vi "Autonomous Independent.vi"() -> ()   [LabVIEW 2016]
doc: "This VI is called when autonomous begins, and will automatically be terminated when autonomous ends. You can carry out timed or sensor driven robot movement independently without needing to return to the caller."
uses:
  2_8_17/Auto_Action.ctl
  <vilib>/Rock Robotics/Network Tables/NT Read Number.vi
  2_11_17/Systems/Global 1.vi
panel:
  out "Auto Mode":dbl=7.0
  in  "Auton_Modes":T2(array[cluster])=[{"Actions"=[{"Effort"=0.55, "Duration"=3.5, "Action"=enum."Nothing", "Encoder"=0.0, "Condition"=FALSE}, {"Effort"=0.0, "Duration"=0.0, "Action"=enum."Nothing", "Encoder"=0.0, "Condition"=FALSE}]}, {"Actions"=[{"Effort"=0.0, "Duration"=0.1, "Action"=enum."Gear1", "Encoder"=6.462, "Condition"=FALSE}, {"Effort"=0.0, "Duration"=0.1, "Action"=enum."Nothing", "Encoder"=0.0, "Condition"=FALSE}, {"Effort"=0.25, "Duration"=1.0, "Action"=enum."Nothing", "Encoder"=38.0, "Condition"=FALSE}, {"Effort"=0.0, "Duration"=0.1, "Action"=enum."Nothing", "Encoder"=0.0, "Condition"=FALSE}, {"Effort"=0.25, "Duration"=0.0, "Action"=enum."Nothing", "Encoder"=57.0, "Condition"=FALSE}, {"Effort"=-0.25, "Duration"=0.0, "Action"=enum."Nothing", "Encoder"=0.0, "Condition"=FALSE}, {"Effort"=1.0, "Duration"=0.0, "Action"=enum."Nothing", "Encoder"=0.0, "Condition"=FALSE}, {"Effort"=0.25, "Duration"=0.0, "Action"=enum."Nothing", "Encoder"=0.0, "Condition"=FALSE}]}, {"Actions"=[{"Effort"=0.0, "Duration"=0.1, "Action"=enum."Drive Encoder Reset", "Encoder"=0.0, "Condition"=FALSE}, {"Effort"=0.0, "Duration"=1.0, "Action"=enum."Gyro Reset", "Encoder"=0.0, "Condition"=FALSE}, {"Effort"=0.3, "Duration"=2.0, "Action"=enum."Drive", "Encoder"=88.0, "Condition"=TRUE}, {"Effort"=1.0, "Duration"=1.0, "Action"=enum."Gear0", "Encoder"=0.0, "Condition"=FALSE}, {"Effort"=1.0, "Duration"=1.0, "Action"=enum."Gear0", "Encoder"=0.0, "Condition"=FALSE}, {"Effort"=1.0, "Duration"=0.5, "Action"=enum."Nothing", "Encoder"=0.0, "Condition"=FALSE}, {"Effort"=0.0, "Duration"=0.0, "Action"=enum."Drive Encoder Reset", "Encoder"=0.0, "Condition"=FALSE}, {"Effort"=0.3, "Duration"=0.5, "Action"=enum."Nothing", "Encoder"=24.0, "Condition"=TRUE}, {"Effort"=0.0, "Duration"=0.0, "Action"=enum."Nothing", "Encoder"=0.0, "Condition"=FALSE}, {"Effort"=-0.2, "Duration"=0.75, "Action"=enum."Drive", "Encoder"=24.0, "Condition"=FALSE}, {"Effort"=0.0, "Duration"=0.0, "Action"=enum."Drive Encoder Reset", "Encoder"=0.0, "Condition"=FALSE}, {"Effort"=-0.25, "Duration"=0.0, "Action"=enum."Nothing", "Encoder"=12.0, "Condition"=FALSE}]}, {"Actions"=[{"Effort"=0.0, "Duration"=0.1, "Action"=enum."Drive Encoder Reset", "Encoder"=6.462, "Condition"=FALSE}, {"Effort"=0.0, "Duration"=0.1, "Action"=enum."Gyro Reset", "Encoder"=0.0, "Condition"=FALSE}, {"Effort"=-0.25, "Duration"=1.0, "Action"=enum."Drive", "Encoder"=6.462, "Condition"=FALSE}, {"Effort"=0.0, "Duration"=0.1, "Action"=enum."Gyro Reset", "Encoder"=0.0, "Condition"=FALSE}, {"Effort"=-0.25, "Duration"=0.0, "Action"=enum."Turn", "Encoder"=57.0, "Condition"=FALSE}, {"Effort"=-0.25, "Duration"=0.0, "Action"=enum."Drive", "Encoder"=7.5, "Condition"=FALSE}, {"Effort"=-1.0, "Duration"=0.0, "Action"=enum."Gear0", "Encoder"=0.0, "Condition"=FALSE}, {"Effort"=0.25, "Duration"=0.0, "Action"=enum."Drive", "Encoder"=3.0, "Condition"=FALSE}]}, {"Actions"=[{"Effort"=0.0, "Duration"=0.1, "Action"=enum."Drive Encoder Reset", "Encoder"=6.462, "Condition"=FALSE}, {"Effort"=0.0, "Duration"=0.1, "Action"=enum."Gyro Reset", "Encoder"=0.0, "Condition"=FALSE}, {"Effort"=-0.25, "Duration"=1.0, "Action"=enum."Drive", "Encoder"=6.462, "Condition"=FALSE}, {"Effort"=0.0, "Duration"=0.1, "Action"=enum."Gyro Reset", "Encoder"=0.0, "Condition"=FALSE}, {"Effort"=-0.25, "Duration"=0.0, "Action"=enum."Turn", "Encoder"=57.0, "Condition"=FALSE}, {"Effort"=-0.25, "Duration"=0.0, "Action"=enum."Drive", "Encoder"=7.5, "Condition"=FALSE}, {"Effort"=-1.0, "Duration"=0.0, "Action"=enum."Gear0", "Encoder"=0.0, "Condition"=FALSE}, {"Effort"=0.25, "Duration"=0.0, "Action"=enum."Drive", "Encoder"=3.0, "Condition"=FALSE}]}, {"Actions"=[{"Effort"=0.0, "Duration"=0.1, "Action"=enum."Drive Encoder Reset", "Encoder"=0.0, "Condition"=FALSE}, {"Effort"=0.0, "Duration"=0.1, "Action"=enum."Gyro Reset", "Encoder"=0.0, "Condition"=FALSE}, {"Effort"=0.25, "Duration"=1.0, "Action"=enum."Drive", "Encoder"=6.462, "Condition"=FALSE}, {"Effort"=1.0, "Duration"=0.1, "Action"=enum."Gyro Reset", "Encoder"=0.0, "Condition"=FALSE}, {"Effort"=0.25, "Duration"=0.0, "Action"=enum."Turn", "Encoder"=57.0, "Condition"=FALSE}, {"Effort"=0.25, "Duration"=0.0, "Action"=enum."Drive", "Encoder"=7.5, "Condition"=FALSE}, {"Effort"=1.0, "Duration"=0.0, "Action"=enum."Gear0", "Encoder"=0.0, "Condition"=FALSE}, {"Effort"=-0.25, "Duration"=0.0, "Action"=enum."Drive", "Encoder"=3.0, "Condition"=FALSE}]}, {"Actions"=[{"Effort"=0.0, "Duration"=0.1, "Action"=enum."Drive Encoder Reset", "Encoder"=0.0, "Condition"=FALSE}, {"Effort"=0.0, "Duration"=0.1, "Action"=enum."Gyro Reset", "Encoder"=0.0, "Condition"=FALSE}, {"Effort"=0.25, "Duration"=5.0, "Action"=enum."Drive", "Encoder"=60000.0, "Condition"=TRUE}, {"Effort"=0.75, "Duration"=1.0, "Action"=enum."Nothing", "Encoder"=0.0, "Condition"=FALSE}, {"Effort"=0.0, "Duration"=1.0, "Action"=enum."Nothing", "Encoder"=0.0, "Condition"=FALSE}, {"Effort"=0.0, "Duration"=0.0, "Action"=enum."Nothing", "Encoder"=0.0, "Condition"=FALSE}]}, {"Actions"=[{"Effort"=0.0, "Duration"=0.5, "Action"=enum."Drive Encoder Reset", "Encoder"=0.0, "Condition"=FALSE}, {"Effort"=0.55, "Duration"=4.25, "Action"=enum."Gyro Reset", "Encoder"=0.0, "Condition"=FALSE}, {"Effort"=0.3, "Duration"=0.0, "Action"=enum."Drive", "Encoder"=60.0, "Condition"=FALSE}, {"Effort"=0.25, "Duration"=1.5, "Action"=enum."Turn", "Encoder"=0.0, "Condition"=FALSE}, {"Effort"=0.25, "Duration"=2.0, "Action"=enum."Vision Correction", "Encoder"=76.6, "Condition"=FALSE}, {"Effort"=0.3, "Duration"=0.5, "Action"=enum."Drive", "Encoder"=0.0, "Condition"=TRUE}]}, {"Actions"=[{"Effort"=0.0, "Duration"=0.0, "Action"=enum."Nothing", "Encoder"=0.0, "Condition"=FALSE}]}]
  # "Nothing"
  # "Boiler Right Right side gear"
  # "Middle Gear"
  # "Boiler Right Left Side Gear"
  # "Boiler Left RightSide Gear"
  # "Boiler Left Left Side Gear"
  # "Drive"
  # "Vision Correction"
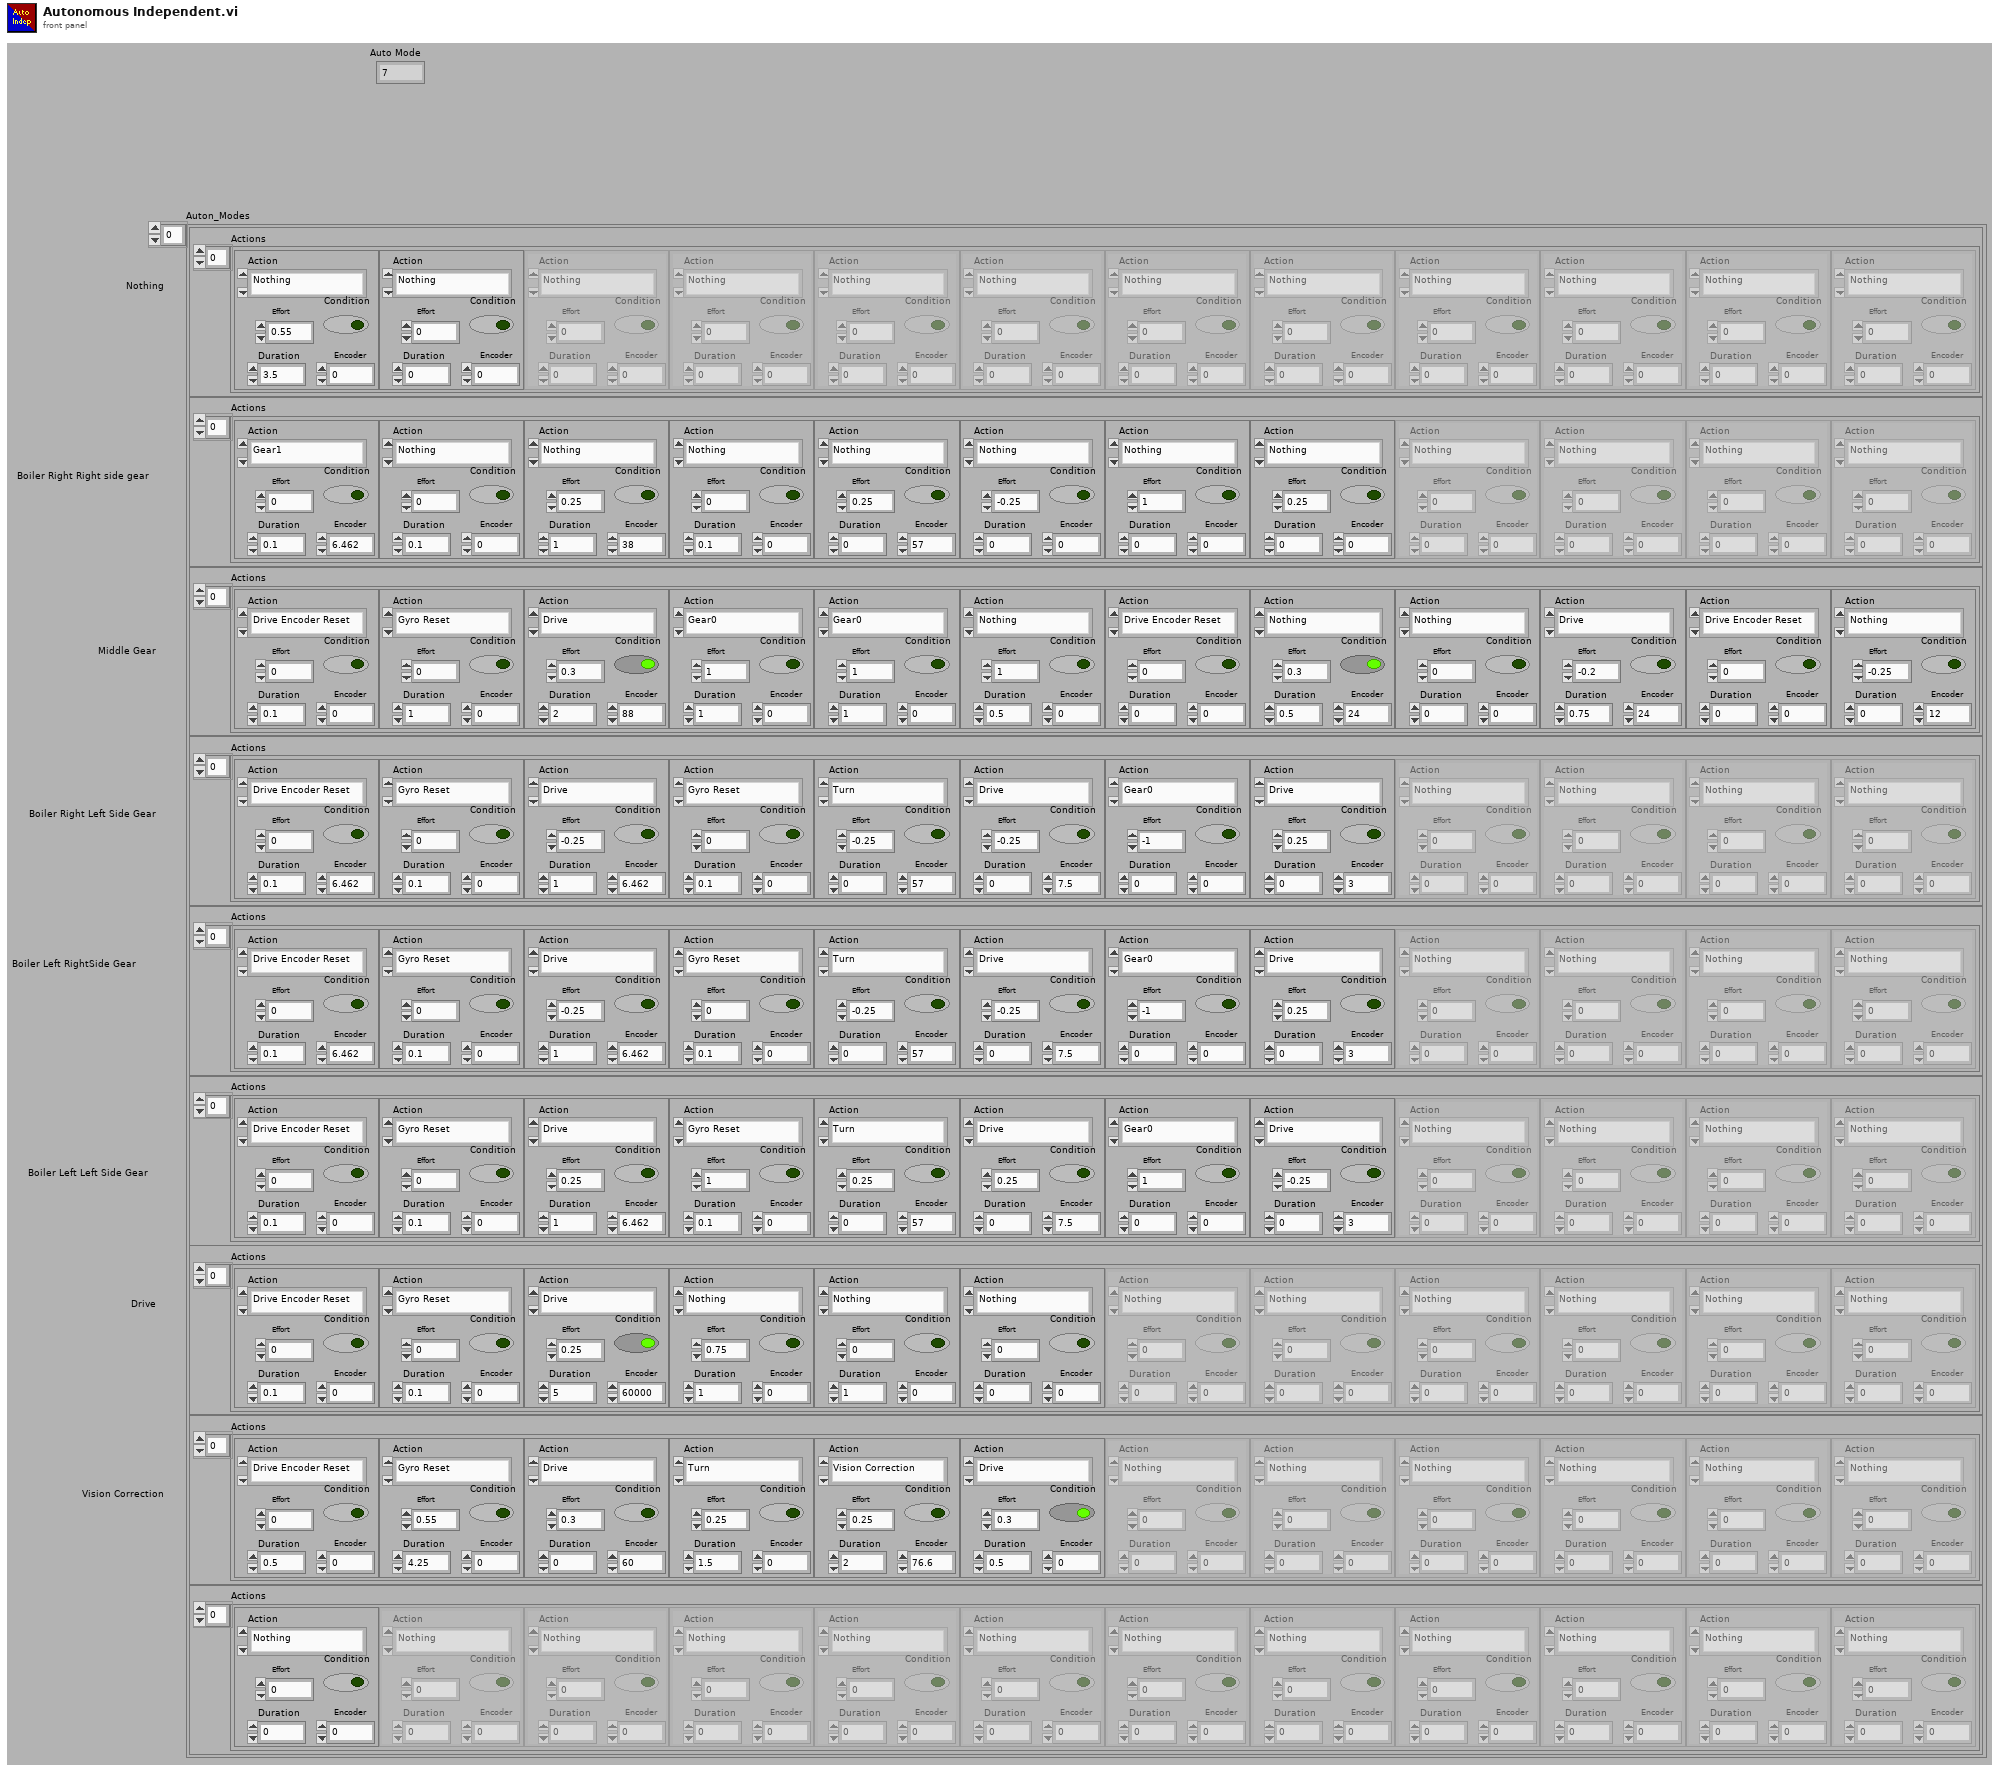
[diagram p1: front panel]
types:
  T1 = typedef "Auto_Action.ctl" = enum16{"Nothing", "Drive", "Vision Correction", "Turn", "Gear0", "Gear1", "Climb", "Intake", "Index", "Shoot", "Test", "Drive Encoder Reset", "Gyro Reset"}
  T2 = cluster{"Actions":cluster{"Effort":dbl, "Duration":dbl, "Action":T1, "Encoder":dbl, "Condition":bool}[]}[]
  T3 = cluster{"Actions":cluster{"Effort":dbl, "Duration":dbl, "Action":T1, "Encoder":dbl, "Condition":bool}[]}
  T4 = cluster{"Effort":dbl, "Duration":dbl, "Action":T1, "Encoder":dbl, "Condition":bool}[]
  T5 = typedef "WPI_MotorControlDeviceRef.ctl" = cluster{"DeviceStatus":errorcluster, "Type":T6, "PWM":cluster{"PWM Channel":T7, "DeadBand":T8}, "CAN":cluster{"Device Number":u8, "SetOutput VI Ref":variant, "GetOutput VI Ref":variant, "Enable VI Ref":variant, "Disable VI Ref":variant, "Data":variant}, "Invert":bool}
  T6 = typedef "WPI_MotorControlType.ctl" = enum16{"PWM", "CAN"}
  T7 = typedef "FPGA_DIOPWMChannel.ctl" = enum8{"PWM 0", "PWM 1", "PWM 2", "PWM 3", "PWM 4", "PWM 5", "PWM 6", "PWM 7", "PWM 8", "PWM 9", "PWM MXP 0", "PWM MXP 1", "PWM MXP 2", "PWM MXP 3", "PWM MXP 4", "PWM MXP 5", "PWM MXP 6", "PWM MXP 7", "PWM MXP 8", "PWM MXP 9", "Invalid"}
  T8 = typedef "WPI_PWMDeadband.ctl" = cluster{"Name":string, "maxPositivePwm":i32, "minPositivePwm":i32, "centerPwm":i32, "maxNegativePwm":i32, "minNegativePwm":i32, "angularRange":u16}
  T9 = typedef "WPI_CANTalonSRX_GlobalStatus.ctl" = cluster{"Applied Throttle":dbl, "Module Enabled":bool, "CAN Error":errorcluster, "Closed Loop Error":dbl, "Forward Limit Switch Closed":bool, "Reverse Limit Switch Closed":bool, "Sensor Position":dbl, "Sensor Velocity":dbl, "Current":dbl, "Sticky Fault - Over Temp":bool, "Sticky Fault - Under Voltage":bool, "Sticky Fault - Forward Limit":bool, "Sticky Fault - Reverse Limit":bool, "Sticky Fault - Forward Soft Limit":bool, "Sticky Fault - Reverse Soft Limit":bool, "Brake is Enabled":bool, "Encoder Position":dbl, "Encoder Velocity":dbl, "Encoder Index Count":dbl, "Encoder A Pin State":bool, "Encoder B Pin State":bool, "Encoder Index Pin State":bool, "Analog In":dbl, "Analog In Velocity":dbl, "Temperature (C)":dbl, "Battery Voltage":dbl, "Control 5 Is Supported":bool, "Current Profile Slot Select":dbl, "Pos Div 8":bool, "Vel Div 4":bool, "Pulse Width Position":i32, "Pulse Width Velocity":i32, "Pulse Width Rise To Rise (us)":i32, "Pulse Width Rise To Fall (us)":i32, "Mot Prof Active Is Under Run":bool, "Mot Prof Active Has Under Run":bool, "Mot Prof Active Is Last":bool, "Mot Prof Active Velocity Only":bool, "Mot Prof Active Is Valid":bool, "Mot Prof Buffer Is Full":bool, "Mot Prof Active Profile Slot Select":i32, "Mot Prof NextID":i32, "Mot Prof Count":i32, "Mot Prof Active Velocity":dbl, "Mot Prof Active Position":dbl, "Mot Prof Output Enable":i32}
  T10 = typedef "WPI_GyroDevRef.ctl" = cluster{"DevStatus":errorcluster, "Analog Channel":T11, "Offset":dbl, "Gain (VoltsPerDegree/Second)":dbl, "Gyro Type":enum16{"Analog", "XRS450"}, "Handle":i32, "SPI Bus":T12, "Device Found":bool, "Sample Rate":dbl, "Calibrate On Open":bool}
  T11 = typedef "FPGA_AIChannel.ctl" = enum8{"AI 0", "AI 1", "AI 2", "AI 3", "AI MXP 0", "AI MXP 1", "AI MXP 2", "AI MXP 3", "Invalid"}
  T12 = typedef "spi_bus.ctl" = enum16{"SPI On-Board, CS0", "SPI On-Board, CS1", "SPI On-Board, CS2", "SPI On-Board, CS3", "SPI MXP", "Invalid"}
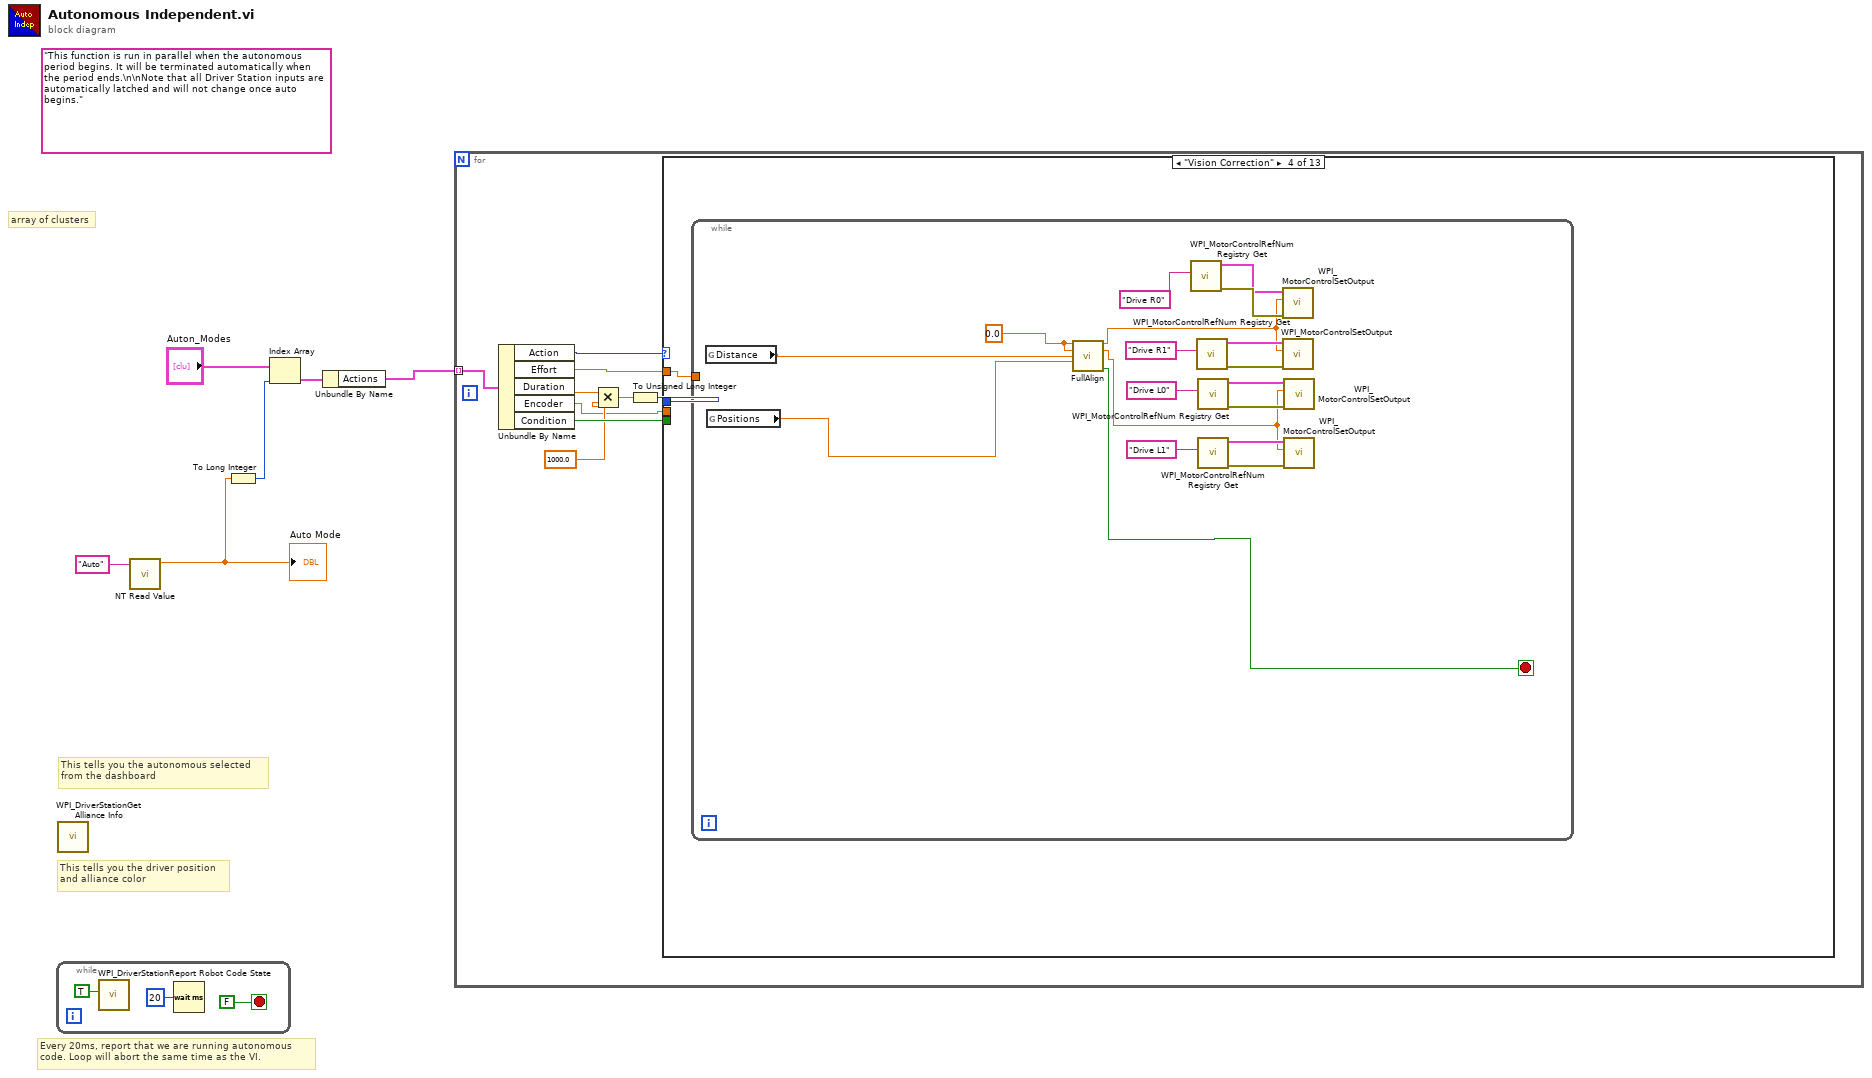
[diagram p0: block diagram]
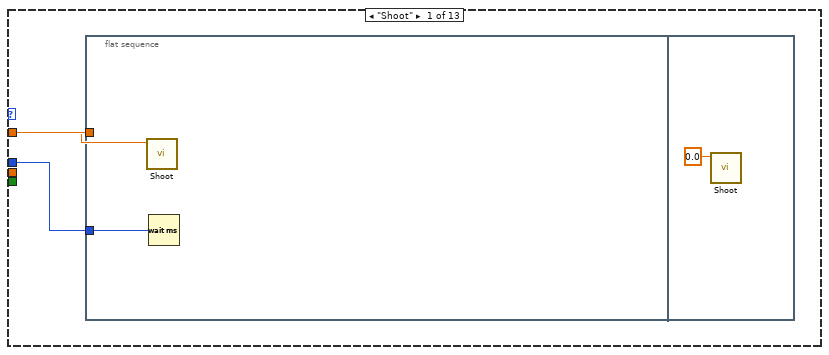
[diagram p2: hidden frame]
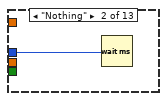
[diagram p3: hidden frame]
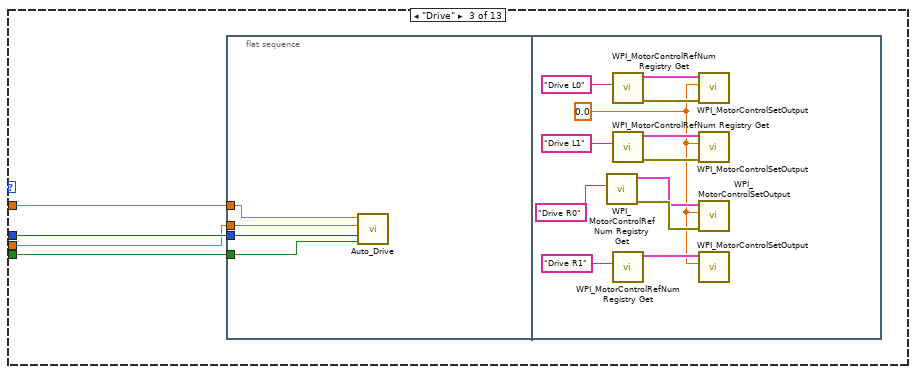
[diagram p4: hidden frame]
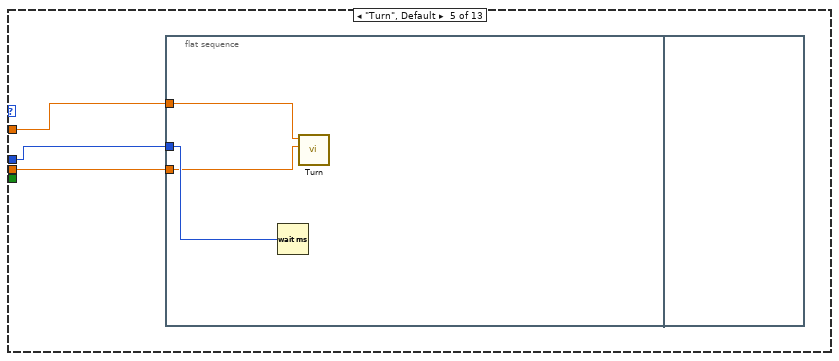
[diagram p5: hidden frame]
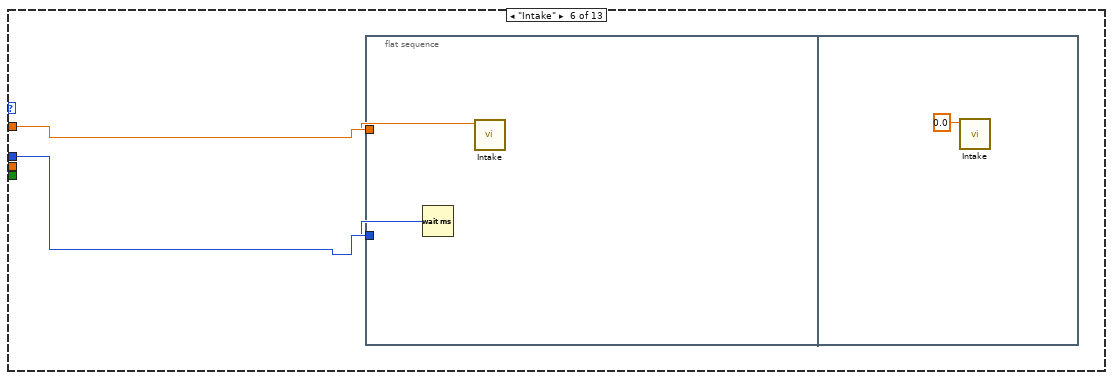
[diagram p6: hidden frame]
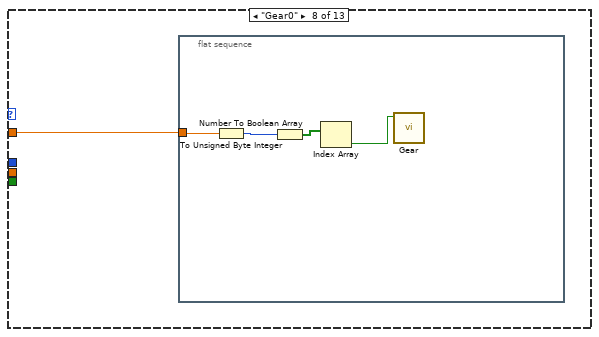
[diagram p8: hidden frame]
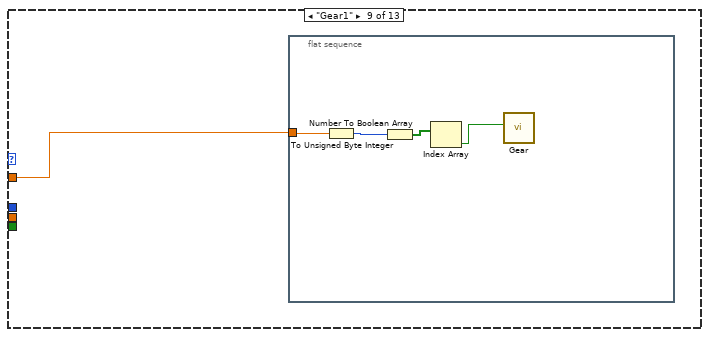
[diagram p9: hidden frame]
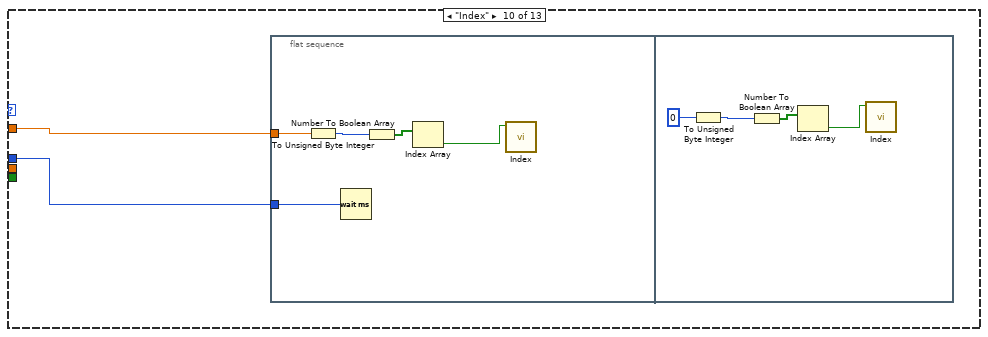
[diagram p10: hidden frame]
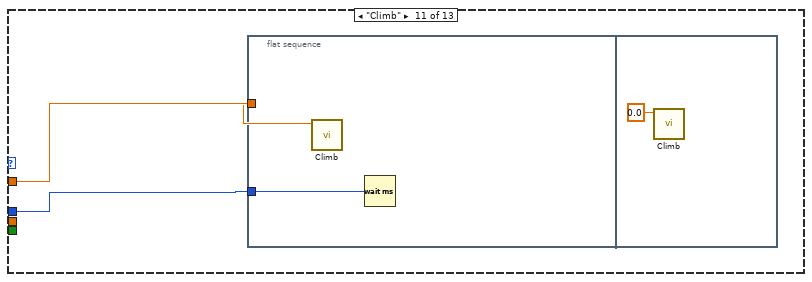
[diagram p11: hidden frame]
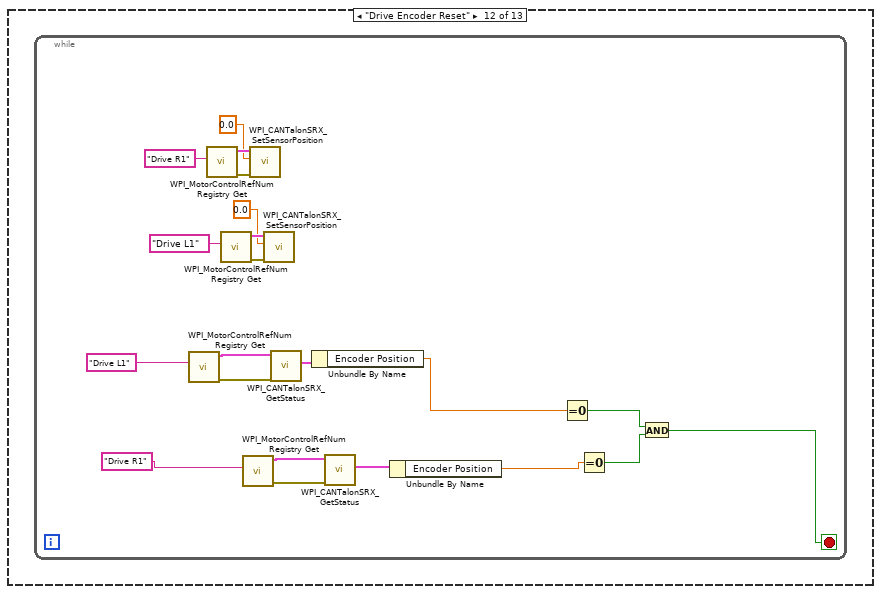
[diagram p12: hidden frame]
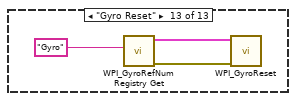
[diagram p13: hidden frame]
diagram:
  (unwired) "This function is run in parallel when the autonomous period begins. It will be terminated automatically when the period ends.\n\nNote that all Driver Station inputs are automatically latched and will not change once auto begins."
  # "This tells you the autonomous selected\nfrom the dashboard"
  # "array of clusters"
  # "Every 20ms, report that we are running autonomous\ncode. Loop will abort the same time as the VI."
  # "This tells you the driver position\nand alliance color"
  n1 = while {
    stop <- FALSE stop-if-true
    n2 = call <vilib>:"WPI_DriverStationReport Robot Code State.vi"("Autonomous"=TRUE) -> ()  [unwired: 10 in, 1 out]
    n3 = Wait (ms)(milliseconds to wait=u32 20) -> ()  [unwired: 1 out]
  }
  n4 = call <vilib>:"WPI_DriverStationGet Alliance Info.vi"() -> ()  [unwired: 12 out]
  n5 = call-poly <vilib>:"NT Read Value.vi"("Name"="Auto") -> ("Numeric"=w1:dbl)  [unwired: 9 in, 1 out]
  "Auto Mode" <- w1
  n6 = To Long Integer(number=w1) -> (32bit integer=w3:i32)
  n7 = Index Array(array="Auton_Modes", index=w3) -> (element=w5:T3)
  n8 = Unbundle By Name(w5) -> ("Actions"=w6:T4)
  n9 = for {
    tunnel: w6 -> [w18] mode=indexing
    n10 = Unbundle By Name(w18) -> ("Action"=w17:T1, "Effort"=w16:dbl, "Duration"=w15:dbl, "Encoder"=w10:dbl, "Condition"=w12:bool)
    n11 = Multiply(x=w15, y=1000.0) -> (x*y=w14:dbl)
    n12 = To Unsigned Long Integer(number=w14) -> (unsigned 32bit integer=w13:u32)
    n13 = case shown="\"Vision Correction\"" w17 {
      tunnel: w16 -> [w20 _ w28 w45 w66 w71 _ w75 w80 w85 w97 _ _]
      tunnel: w13 -> [w19 w24 w27 _ w65 w70 _ _ _ w86 w96 _ _]
      tunnel: w12 -> [_ _ w26 _ _ _ _ _ _ _ _ _ _]
      tunnel: w10 -> [_ _ w25 _ w64 _ _ _ _ _ _ _ _]
      frame "Shoot" {
        n14 = flat-sequence {
          tunnel: w20 -> [w22]
          tunnel: w19 -> [w21]
          frame #0 {
            n15 = call "Shoot.vi"("Set RPM"=w22) -> ()  [unwired: 11 in]
            n16 = Wait (ms)(milliseconds to wait=w21) -> ()  [unwired: 1 out]
          }
          frame #1 {
            n17 = call "Shoot.vi"("Set RPM"=0.0 ("Effort")) -> ()  [unwired: 11 in]
          }
        }
      }
      frame "Nothing" {
        n18 = Wait (ms)(milliseconds to wait=w24) -> ()  [unwired: 1 out]
      }
      frame "Drive" {
        n19 = flat-sequence {
          tunnel: w28 -> [w32]
          tunnel: w27 -> [w31]
          tunnel: w26 -> [w30]
          tunnel: w25 -> [w29]
          frame #0 {
            n20 = call "Auto_Drive.vi"("Timer?"=w30, "Duration"=w31, "distance"=w29, "Drive Effort"=w32) -> ()  [unwired: 8 in]
          }
          frame #1 {
            w33 = 0.0 ("Drive L")
            n21 = call <vilib>:"WPI_MotorControlRefNum Registry Get.vi"("refnum name"="Drive R0") -> ("error out"=w38:errorcluster, "MotorControlDevRef"=w34:T5)  [unwired: 9 in]
            n22 = call <vilib>:"WPI_MotorControlRefNum Registry Get.vi"("refnum name"="Drive L0") -> ("error out"=w39:errorcluster, "MotorControlDevRef"=w40:T5)  [unwired: 9 in]
            n23 = call <vilib>:"WPI_MotorControlRefNum Registry Get.vi"("refnum name"="Drive L1") -> ("error out"=w43:errorcluster, "MotorControlDevRef"=w42:T5)  [unwired: 9 in]
            n24 = call <vilib>:"WPI_MotorControlRefNum Registry Get.vi"("refnum name"="Drive R1") -> ("MotorControlDevRef"=w36:T5)  [unwired: 9 in, 1 out]
            n25 = call <vilib>:"WPI_MotorControlSetOutput.vi"("error in (no error)"=w39, "Output"=w33, "MotorControlDevRef"=w40) -> ()  [unwired: 6 in, 3 out]
            n26 = call <vilib>:"WPI_MotorControlSetOutput.vi"("error in (no error)"=w43, "Output"=w33, "MotorControlDevRef"=w42) -> ()  [unwired: 6 in, 3 out]
            n27 = call <vilib>:"WPI_MotorControlSetOutput.vi"("error in (no error)"=w38, "Output"=w33, "MotorControlDevRef"=w34) -> ()  [unwired: 6 in, 3 out]
            n28 = call <vilib>:"WPI_MotorControlSetOutput.vi"("Output"=w33, "MotorControlDevRef"=w36) -> ()  [unwired: 7 in, 3 out]
          }
        }
      }
      frame "Vision Correction" {
        n29 = while {
          tunnel: w45 -> [_]
          stop <- w46 stop-if-true
          w49 = 0.0
          n30 = global read "Global 1.vi" "Distance"() -> (w48:dbl)
          n31 = global read "Global 1.vi" "Positions"() -> (w47:dbl)
          n32 = call "FullAlign.vi"("Joystick 0"=w49, "Joystick 1"=w49, "Distance"=w48, "Angle"=w47) -> ("Right Motor"=w51:dbl, "Left Motor"=w50:dbl, "In Range?"=w46:bool)  [unwired: 9 in]
          n33 = call <vilib>:"WPI_MotorControlRefNum Registry Get.vi"("refnum name"="Drive R0") -> ("error out"=w57:errorcluster, "MotorControlDevRef"=w53:T5)  [unwired: 9 in]
          n34 = call <vilib>:"WPI_MotorControlRefNum Registry Get.vi"("refnum name"="Drive R1") -> ("error out"=w52:errorcluster, "MotorControlDevRef"=w55:T5)  [unwired: 9 in]
          n35 = call <vilib>:"WPI_MotorControlRefNum Registry Get.vi"("refnum name"="Drive L0") -> ("error out"=w58:errorcluster, "MotorControlDevRef"=w59:T5)  [unwired: 9 in]
          n36 = call <vilib>:"WPI_MotorControlRefNum Registry Get.vi"("refnum name"="Drive L1") -> ("error out"=w62:errorcluster, "MotorControlDevRef"=w61:T5)  [unwired: 9 in]
          n37 = call <vilib>:"WPI_MotorControlSetOutput.vi"("error in (no error)"=w57, "Output"=w51, "MotorControlDevRef"=w53) -> ()  [unwired: 6 in, 3 out]
          n38 = call <vilib>:"WPI_MotorControlSetOutput.vi"("error in (no error)"=w52, "Output"=w51, "MotorControlDevRef"=w55) -> ()  [unwired: 6 in, 3 out]
          n39 = call <vilib>:"WPI_MotorControlSetOutput.vi"("error in (no error)"=w58, "Output"=w50, "MotorControlDevRef"=w59) -> ()  [unwired: 6 in, 3 out]
          n40 = call <vilib>:"WPI_MotorControlSetOutput.vi"("error in (no error)"=w62, "Output"=w50, "MotorControlDevRef"=w61) -> ()  [unwired: 6 in, 3 out]
        }
      }
      frame "Turn", Default {
        n41 = flat-sequence {
          tunnel: w66 -> [w69]
          tunnel: w65 -> [w68]
          tunnel: w64 -> [w67]
          frame #0 {
            n42 = Wait (ms)(milliseconds to wait=w68) -> ()  [unwired: 1 out]
            n43 = call "Turn.vi"("Target"=w67, "Effort"=w69) -> ()  [unwired: 10 in]
          }
          frame #1 {
          }
        }
      }
      frame "Intake" {
        n44 = flat-sequence {
          tunnel: w71 -> [w73]
          tunnel: w70 -> [w72]
          frame #0 {
            n45 = Wait (ms)(milliseconds to wait=w72) -> ()  [unwired: 1 out]
            n46 = call "Intake.vi"("Effort"=w73) -> ()  [unwired: 11 in]
          }
          frame #1 {
            n47 = call "Intake.vi"("Effort"=0.0) -> ()  [unwired: 11 in]
          }
        }
      }
      frame "Test" {
      }
      frame "Gear0" {
        n48 = flat-sequence {
          tunnel: w75 -> [w79]
          frame #0 {
            n49 = To Unsigned Byte Integer(number=w79) -> (unsigned 8bit integer=w78:u8)
            n50 = Number To Boolean Array(number=w78) -> (Boolean array=w77:bool[])
            n51 = Index Array(array=w77) -> (element=w76:bool)  [unwired: 1 in]
            n52 = call "Gear.vi"("Gear0?"=w76) -> ()  [unwired: 11 in]
          }
        }
      }
      frame "Gear1" {
        n53 = flat-sequence {
          tunnel: w80 -> [w84]
          frame #0 {
            n54 = To Unsigned Byte Integer(number=w84) -> (unsigned 8bit integer=w83:u8)
            n55 = Number To Boolean Array(number=w83) -> (Boolean array=w82:bool[])
            n56 = Index Array(array=w82) -> (element=w81:bool)  [unwired: 1 in]
            n57 = call "Gear.vi"("Gear1?"=w81) -> ()  [unwired: 11 in]
          }
        }
      }
      frame "Index" {
        n58 = flat-sequence {
          tunnel: w86 -> [w88]
          tunnel: w85 -> [w87]
          frame #0 {
            n59 = To Unsigned Byte Integer(number=w87) -> (unsigned 8bit integer=w91:u8)
            n60 = Wait (ms)(milliseconds to wait=w88) -> ()  [unwired: 1 out]
            n61 = Number To Boolean Array(number=w91) -> (Boolean array=w90:bool[])
            n62 = Index Array(array=w90) -> (element=w89:bool)  [unwired: 1 in]
            n63 = call "Index.vi"("Index?"=w89) -> ()  [unwired: 11 in]
          }
          frame #1 {
            n64 = To Unsigned Byte Integer(number=u8 0) -> (unsigned 8bit integer=w94:u8)
            n65 = Number To Boolean Array(number=w94) -> (Boolean array=w95:bool[])
            n66 = Index Array(array=w95) -> (element=w92:bool)  [unwired: 1 in]
            n67 = call "Index.vi"("Index?"=w92) -> ()  [unwired: 11 in]
          }
        }
      }
      frame "Climb" {
        n68 = flat-sequence {
          tunnel: w97 -> [w99]
          tunnel: w96 -> [w98]
          frame #0 {
            n69 = call "Climb.vi"("Effort"=w99) -> ()  [unwired: 11 in]
            n70 = Wait (ms)(milliseconds to wait=w98) -> ()  [unwired: 1 out]
          }
          frame #1 {
            n71 = call "Climb.vi"("Effort"=0.0) -> ()  [unwired: 11 in]
          }
        }
      }
      frame "Drive Encoder Reset" {
        n72 = while {
          stop <- w101 stop-if-true
          n73 = call <vilib>:"WPI_MotorControlRefNum Registry Get.vi"("refnum name"="Drive L1") -> ("error out"=w111:errorcluster, "MotorControlDevRef"=w106:T5)  [unwired: 9 in]
          n74 = call <vilib>:"WPI_MotorControlRefNum Registry Get.vi"("refnum name"="Drive R1") -> ("error out"=w116:errorcluster, "MotorControlDevRef"=w115:T5)  [unwired: 9 in]
          n75 = call <vilib>:"WPI_MotorControlRefNum Registry Get.vi"("refnum name"="Drive L1") -> ("error out"=w118:errorcluster, "MotorControlDevRef"=w119:T5)  [unwired: 9 in]
          n76 = call <vilib>:"WPI_MotorControlRefNum Registry Get.vi"("refnum name"="Drive R1") -> ("error out"=w108:errorcluster, "MotorControlDevRef"=w107:T5)  [unwired: 9 in]
          n77 = call <vilib>:"WPI_CANTalonSRX_SetSensorPosition.vi"("error in (no error)"=w116, "New Sensor Position"=0.0, "CAN Talon SRX Ref"=w115) -> ()  [unwired: 7 in, 2 out]
          n78 = call <vilib>:"WPI_CANTalonSRX_SetSensorPosition.vi"("error in (no error)"=w118, "New Sensor Position"=0.0, "CAN Talon SRX Ref"=w119) -> ()  [unwired: 7 in, 2 out]
          n79 = call <vilib>:"WPI_CANTalonSRX_GetStatus.vi"("error in (no error)"=w111, "CAN Talon SRX Ref"=w106) -> ("Talon SRX Status"=w109:T9)  [unwired: 7 in, 2 out]
          n80 = Unbundle By Name(w109) -> ("Encoder Position"=w104:dbl)
          n81 = call <vilib>:"WPI_CANTalonSRX_GetStatus.vi"("error in (no error)"=w108, "CAN Talon SRX Ref"=w107) -> ("Talon SRX Status"=w110:T9)  [unwired: 7 in, 2 out]
          n82 = Unbundle By Name(w110) -> ("Encoder Position"=w105:dbl)
          n83 = Equal To 0?(x=w104) -> (x = 0?=w103:bool)
          n84 = Equal To 0?(x=w105) -> (x = 0?=w102:bool)
          n85 = And(x=w103, y=w102) -> (x .and. y?=w101:bool)
        }
      }
      frame "Gyro Reset" {
        n86 = call <vilib>:"WPI_GyroRefNum Registry Get.vi"("refnum name"="Gyro") -> ("error out"=w123:errorcluster, "GyroDevRef"=w124:T10)  [unwired: 9 in]
        n87 = call <vilib>:"WPI_GyroReset.vi"("error in"=w123, "GyroDevRef"=w124) -> ()  [unwired: 8 in, 2 out]
      }
    }
  }
